vi "createDcimgFilename.vi"(1 "origPath":path) -> (0 "dcimgPath":path)   [LabVIEW 2015]
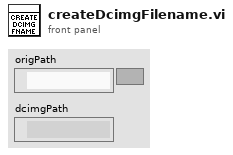
[diagram p1: front panel]
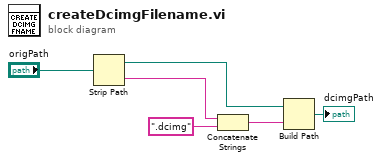
[diagram p0: block diagram]
diagram:
  n1 = Strip Path(path="origPath") -> (stripped path=w2:path, name=w3:string)
  n2 = Concatenate Strings(w3, ".dcimg" ("name or relative path")) -> (w5:string)
  n3 = Build Path(base path=w2, name or relative path=w5) -> (appended path=→"dcimgPath":path)
